vi "SPARK Start Daemons.vi"(8 "error in (no error)":errorcluster) -> (0 "error out":errorcluster)   [LabVIEW 2023]
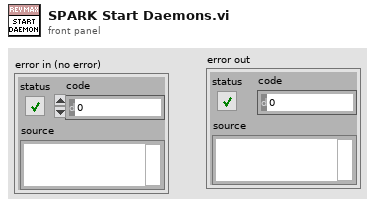
[diagram p1: front panel]
types:
  T1 = enum32{"Bad", "Idle", "Run top level", "Running"}
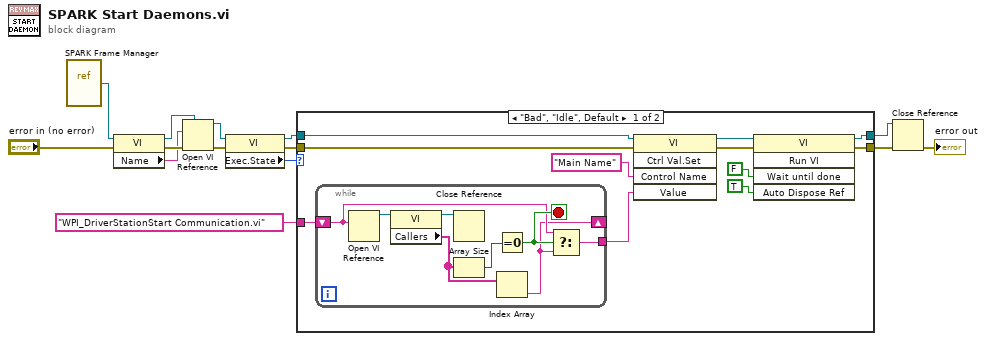
[diagram p0: block diagram]
diagram:
  n1 = vi-ref "SPARK Frame Manager.vi"() -> (w8:refnum<vi>)
  n2 = property class="VI"(reference=w8, error in="error in (no error)") -> (reference out=w9:refnum<vi>, error out=w11:errorcluster, "Name"=w10:string)
  n3 = Open VI Reference(type specifier VI Refnum (for type only)=w9, vi path=w10, error in (no error)=w11) -> (vi reference=w13:refnum<vi>, error out=w12:errorcluster)  [unwired: 3 in]
  n4 = property class="VI"(reference=w13, error in=w12) -> (reference out=w5:refnum<vi>, error out=w6:errorcluster, "Exec.State"=w7:T1)
  n5 = case shown="\"Bad\", \"Idle\", Default" w7 {
    tunnel: w6 -> [w19 w35]
    tunnel: w5 -> [w23 w34]
    tunnel: [w21 w35] -> w4
    tunnel: [w22 w34] -> w3
    tunnel: "WPI_DriverStationStart Communication.vi" -> [w15 _]
    frame "Bad", "Idle", Default {
      n6 = while {
        shift-right: [w28] -> _
        shift-left: w15 -> [w29]
        tunnel: [w27] -> w17
        stop <- w30 stop-if-true
        n7 = Open VI Reference(vi path=w29) -> (vi reference=w33:refnum<vi>)  [unwired: 1 in, 5 out]
        n8 = property class="VI"(reference=w33) -> (reference out=w26:refnum<vi>, "Callers"=w31:string[])  [unwired: 1 in, 1 out]
        n9 = Close Reference(reference=w26) -> ()  [unwired: 1 in, 1 out]
        n10 = Array Size(array=w31) -> (size(s)=w32:i32)
        n11 = Equal To 0?(x=w32) -> (x = 0?=w30:bool)
        n12 = Index Array(array=w31) -> (element=w28:string)  [unwired: 1 in]
        n13 = Select(t=w29, s=w30, f=w28) -> (s? t:f=w27:string)
      }
      n14 = invoke class="VI" method="Ctrl Val.Set"(reference=w23, error in=w19, "Control Name"="Main Name", "Value"=w17) -> (reference out=w20:refnum<vi>, error out=w18:errorcluster)  [unwired: 1 in, 3 out]
      n15 = invoke class="VI" method="Run VI"(reference=w20, error in=w18, "Wait until done"=FALSE ("Wait Until Done"), "Auto Dispose Ref"=TRUE ("Auto Dispose Reference")) -> (reference out=w22:refnum<vi>, error out=w21:errorcluster)  [unwired: 1 in, 3 out]
    }
    frame "Run top level", "Running" {
    }
  }
  n16 = Close Reference(reference=w3, error in (no error)=w4) -> (error out=→"error out":errorcluster)
